vi "CheckAllPreferences.vi"() -> ()   [LabVIEW 2022 SP3]
uses:
  <vilib>/Utility/miscctls.llb/LVRangeTypeDef.ctl
  PreferencesControl.ctl
  Mic/Mic_Global.vi
panel:
  in  "Tab Control":enum32{"Files", "Globlals"}(tab)
  out "description":string
  out "Test Globals":T1
  out "Notes Out":string
  out "DataPath Out":path
  in  "Lists":u16(ring) items=["favorites", "117 vlns by B1 avg HV", "Admittance repeatability", "All 123 vlns group avg", "Internal mic 20920 ", "IVCI 18 all H adm rad", "ivci18 top 13 Adm H.AvR", "IVCI18 top 13 rad. H avg", "Mic distance B", "Mic distance test H12", "New York HV", "Paris 12 HV", "Rubio 6 spherical equatorial", "Some favorites 2018-2021", "String tension experiment", "Violas"]
  out "FRF settings":cluster{"XScale.Range":T2, "YScale.Range":T2}
  out "View":T3={"Alerts"=FALSE, "Log X Axis"=TRUE, "dB scale"=TRUE, "Averaging"=TRUE, "Fade"=0.8181818181818182, "Centroids?"=TRUE, "line thickness"=1}
  out "X Settings":cluster{"X_Low":dbl, "X_High":dbl}
  out "List contents":string
  in  "Templates":u16(ring) items=["", "accelerometer taptone Scratchpad", "Admittance H", "Admittance Scratchpad", "Current Settings", "Internal mic H", "JC Admit H laser", "JC Admit.HV laser", "JC H 12 radiation", "JC H 7 radiation", "JC HV 24 radiation", "Laser Admitance ScratchPad", "Radiation H 1", "Radiation ScratchPad", "ScratchPad", "Tap repeatabilty H20", "TapTones ScratchPad"]
  out "Settings out":T4={"Name of test"="", "Date"=timestamp(0 s since 1904-01-01), "Location"="", "Template"="", "Soundcard"="", "resolution"=32, "Sampling rate"=48000, "Ch1 Gain "=25.0, "Ch2 Gain"=10.0, "Sample time (s)"=0.3, "Pre-trigger (s)"=0.01, "Hammer Threshold"=10.0, "Positions"=12, "Taps/Position"=5, "Set Names"="", "Freq resolution"=10.0, "Hammer cutoff"=0.0, "Mic cutoff"=0.0, "Double bounce "=0.0, "Hammer Cal"=10.0, "dB Offset"=0.0, "Accel Cal"=10.0, "Vibrometer Cal"=0.0, "Mic Cal"=0.0, "Output"=2, "Voltage Cal"=1.0, "Vibrometer Port"="ASRL27::INSTR", "Range"=4, "High Pass"=2, "Bandwidth"=4, "X Range"=[], "Y Range"=[], "dB Spread"=0.0, "Trigger"=0, "Ch_1"=25, "Ch_2"=25, "flip?"=FALSE, "60Hz"=FALSE, "Time offset"=0.0, "Piezo Cal"=1.0, "Default Notes"=""} {"Ch_2" min=1 step=1; "Ch_1" min=1 max=100 step=1; "Trigger" items=["Hammer (force)", "Self-tap", "Spacebar"]; "Bandwidth" items=["1 kHz"=1, "5 kHz"=5, "10 kHz"=10, "25 kHz"=25, "50 kHz"=50, "100 kHz"=100]; "High Pass" items=["Off", "13 Hz", "104 Hz"]; "Range" items=["10 mm/s"=1, "20 mm/s"=2, "50 mm/s"=5, "100 mm/s"=10, "200 mm/s"=20, "500 mm/s"=50, "1 m/s"=100, "2 m/s"=200]; "Output" items=["Accelerometer", "Speed (from acceleration)", "Microphone", "Vibrometer", "Piezo"]; "Voltage Cal" format="%#_13g"; "Ch2 Gain" format="%#_13g"; "Ch1 Gain" format="%#_13g"; "Double bounce" min=0.0; "Mic cutoff" min=0.0 format="%#_4g"; "Hammer cutoff" min=0.0 format="%#_4g"; "Freq resolution" min=0.0; "Pre-trigger (s)" format="%#_13g"; "Date" format="%<%H:%M\n%d/%m/%y>T"; "resolution" items=["16 bit"=16, "24 bit"=24, "32 bit"=32]; "Sampling rate" items=["22050 samp/s"=22050, "44100 samp/s"=44100, "48000 samp/s"=48000]}
  out "comma?":bool
  in  "Cal File":path
  out "DAQ":string="DAQX"
  out "Scratch":string="ScratchPad"
  out "ID":i32[](array[numeric])
  out "View 2":T3={"Alerts"=FALSE, "Log X Axis"=TRUE, "dB scale"=TRUE, "Averaging"=TRUE, "Fade"=0.8181818181818182, "Centroids?"=TRUE, "line thickness"=1}
  out "Version":string="ObieApp 1.1b3"
  out "Settings":T4={"Name of test"="", "Date"=timestamp(3691169924 s since 1904-01-01), "Location"="", "Template"="", "Soundcard"="", "resolution"=32, "Sampling rate"=48000, "Ch1 Gain "=25.0, "Ch2 Gain"=10.0, "Sample time (s)"=0.3, "Pre-trigger (s)"=0.01, "Hammer Threshold"=0.1, "Positions"=12, "Taps/Position"=5, "Set Names"="", "Freq resolution"=1.0, "Hammer cutoff"=0.0, "Mic cutoff"=0.0, "Double bounce "=0.1, "Hammer Cal"=23.6, "dB Offset"=0.0, "Accel Cal"=1.014, "Vibrometer Cal"=1.0, "Mic Cal"=48.5, "Output"=2, "Voltage Cal"=3.8, "Vibrometer Port"="ASRL27::INSTR", "Range"=50, "High Pass"=2, "Bandwidth"=25, "X Range"=[], "Y Range"=[], "dB Spread"=40.0, "Trigger"=0, "Ch_1"=1, "Ch_2"=2, "flip?"=FALSE, "60Hz"=FALSE, "Time offset"=0.0, "Piezo Cal"=1.0, "Default Notes"=""} {"Ch_2" min=1 step=1; "Ch_1" min=1 max=100 step=1; "Trigger" items=["Hammer (force)", "Self-tap", "Spacebar"]; "Bandwidth" items=["1 kHz"=1, "5 kHz"=5, "10 kHz"=10, "25 kHz"=25, "50 kHz"=50, "100 kHz"=100]; "High Pass" items=["Off", "13 Hz", "104 Hz"]; "Range" items=["10 mm/s"=1, "20 mm/s"=2, "50 mm/s"=5, "100 mm/s"=10, "200 mm/s"=20, "500 mm/s"=50, "1 m/s"=100, "2 m/s"=200]; "Output" items=["Accelerometer", "Speed (from acceleration)", "Microphone", "Vibrometer", "Piezo"]; "Voltage Cal" format="%#_13g"; "Ch2 Gain" format="%#_13g"; "Ch1 Gain" format="%#_13g"; "Double bounce" min=0.0; "Mic cutoff" min=0.0 format="%#_4g"; "Hammer cutoff" min=0.0 format="%#_4g"; "Freq resolution" min=0.0; "Pre-trigger (s)" format="%#_13g"; "Date" format="%<%H:%M\n%d/%m/%y>T"; "resolution" items=["16 bit"=16, "24 bit"=24, "32 bit"=32]; "Sampling rate" items=["22050 samp/s"=22050, "44100 samp/s"=44100, "48000 samp/s"=48000]}
  out "Default Settings":T4={"Name of test"="ScratchPad", "Date"=timestamp(0 s since 1904-01-01), "Location"="Home", "Template"="ScratchPad", "Soundcard"="OCTA-CAPTURE", "resolution"=32, "Sampling rate"=48000, "Ch1 Gain "=20.0, "Ch2 Gain"=20.0, "Sample time (s)"=0.3, "Pre-trigger (s)"=0.001, "Hammer Threshold"=0.01, "Positions"=12, "Taps/Position"=5, "Set Names"="H,V", "Freq resolution"=1.0, "Hammer cutoff"=0.025, "Mic cutoff"=0.25, "Double bounce "=0.01, "Hammer Cal"=1.0, "dB Offset"=0.0, "Accel Cal"=1.0, "Vibrometer Cal"=1.0, "Mic Cal"=1.0, "Output"=2, "Voltage Cal"=1.0, "Vibrometer Port"="ASRL27::INSTR", "Range"=50, "High Pass"=2, "Bandwidth"=25, "X Range"=[{"Minimum"=200.0, "Maximum"=10000.0, "Increment"=2500.0, "Minor Increment"=500.0, "Start"=2500.0}, {"Minimum"=0.0, "Maximum"=0.05, "Increment"=0.025, "Minor Increment"=0.0025, "Start"=0.0}, {"Minimum"=0.0, "Maximum"=0.3, "Increment"=0.1, "Minor Increment"=0.01, "Start"=0.0}, {"Minimum"=200.0, "Maximum"=10000.0, "Increment"=10.0, "Minor Increment"=100.0, "Start"=1000.0}], "Y Range"=[{"Minimum"=-25.0, "Maximum"=0.0, "Increment"=5.0, "Minor Increment"=1.0, "Start"=-25.0}, {"Minimum"=-0.1, "Maximum"=1.0, "Increment"=0.25, "Minor Increment"=0.05, "Start"=0.0}, {"Minimum"=-1.0, "Maximum"=1.0, "Increment"=0.5, "Minor Increment"=0.1, "Start"=-1.0}, {"Minimum"=-10.0, "Maximum"=30.0, "Increment"=10.0, "Minor Increment"=0.5, "Start"=-10.0}], "dB Spread"=40.0, "Trigger"=0, "Ch_1"=1, "Ch_2"=2, "flip?"=FALSE, "60Hz"=FALSE, "Time offset"=0.0, "Piezo Cal"=1.0, "Default Notes"=""} {"Ch_2" min=1 step=1; "Ch_1" min=1 max=100 step=1; "Trigger" items=["Hammer (force)", "Self-tap", "Spacebar"]; "Bandwidth" items=["1 kHz"=1, "5 kHz"=5, "10 kHz"=10, "25 kHz"=25, "50 kHz"=50, "100 kHz"=100]; "High Pass" items=["Off", "13 Hz", "104 Hz"]; "Range" items=["10 mm/s"=1, "20 mm/s"=2, "50 mm/s"=5, "100 mm/s"=10, "200 mm/s"=20, "500 mm/s"=50, "1 m/s"=100, "2 m/s"=200]; "Output" items=["Accelerometer", "Speed (from acceleration)", "Microphone", "Vibrometer", "Piezo"]; "Voltage Cal" format="%#_13g"; "Ch2 Gain" format="%#_13g"; "Ch1 Gain" format="%#_13g"; "Double bounce" min=0.0; "Mic cutoff" min=0.0 format="%#_4g"; "Hammer cutoff" min=0.0 format="%#_4g"; "Freq resolution" min=0.0; "Pre-trigger (s)" format="%#_13g"; "Date" format="%<%H:%M\n%d/%m/%y>T"; "resolution" items=["16 bit"=16, "24 bit"=24, "32 bit"=32]; "Sampling rate" items=["22050 samp/s"=22050, "44100 samp/s"=44100, "48000 samp/s"=48000]}
  in  "Last":path
  out "devices":string[](array[string])=["Built-in Microph", "OCTA-CAPTURE"]
  in  "Task":T5(ring)=enum."One Shot - waiting"
  # "Hz"
  # "dB"
  # "dB"
  # "sec"
  # "sec"
  # "mV/Pa"
  # "mV/m/s2"
  # "mV/mm/s"
  # "V/N"
  # "sec"
  # "sec"
  # "mV/N"
  # "a.u."
  # "a.u."
  # "sec"
  # "Microphone"
  # "Labels"
  # "File Info"
  # "Hz"
  # "dB"
  # "dB"
  # "sec"
  # "sec"
  # "mV/Pa"
  # "mV/m/s2"
  # "mV/mm/s"
  # "V/N"
  # "sec"
  # "sec"
  # "mV/N"
  # "a.u."
  # "a.u."
  # "sec"
  # "Hz"
  # "dB"
  # "dB"
  # "sec"
  # "sec"
  # "mV/Pa"
  # "mV/m/s2"
  # "mV/mm/s"
  # "V/N"
  # "sec"
  # "sec"
  # "mV/N"
  # "a.u."
  # "a.u."
  # "sec"
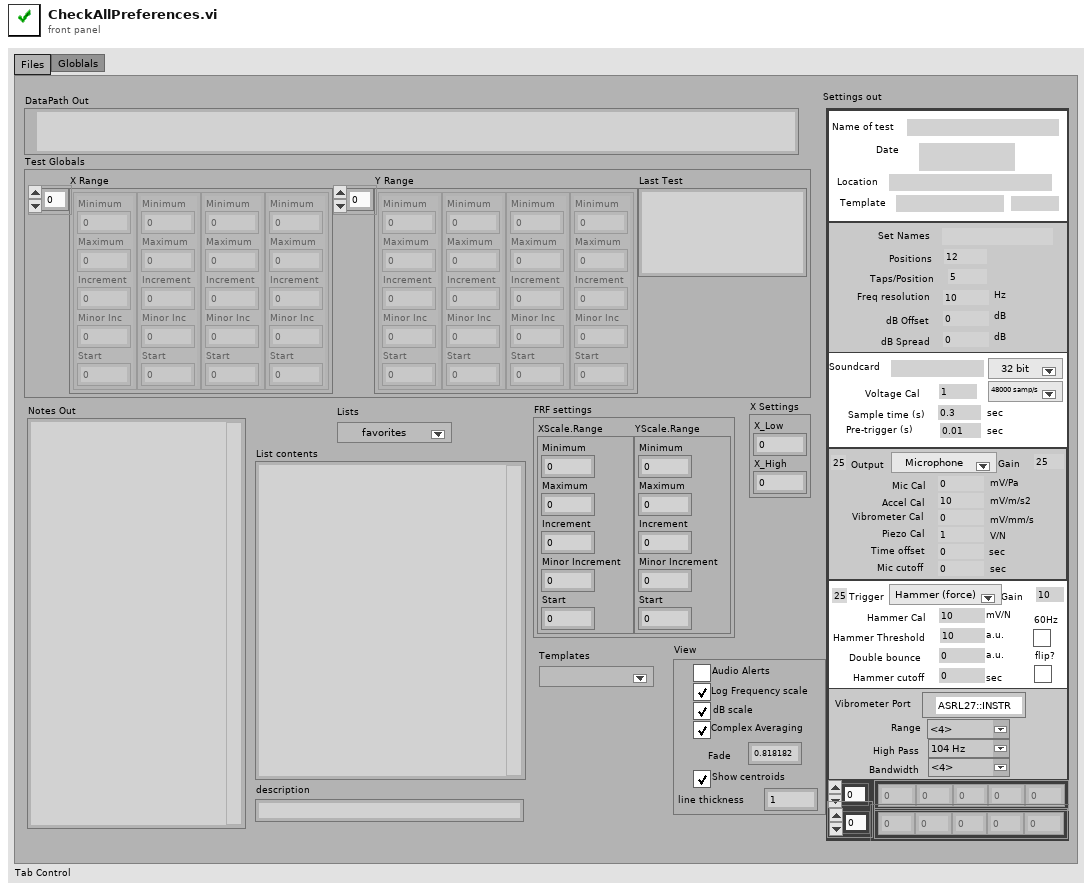
[diagram p1: front panel]
types:
  T1 = cluster{"X Range":cluster{"Minimum":dbl, "Maximum":dbl, "Increment":dbl, "Minor Inc":dbl, "Start":dbl}[], "Y Range":cluster{"Minimum":dbl, "Maximum":dbl, "Increment":dbl, "Minor Inc":dbl, "Start":dbl}[], "Last Test":string}
  T2 = typedef "LVRangeTypeDef.ctl" = cluster{"Minimum":dbl, "Maximum":dbl, "Increment":dbl, "Minor Increment":dbl, "Start":dbl}
  T3 = cluster{"Alerts":bool, "Log X Axis":bool, "dB scale":bool, "Averaging":bool, "Fade":dbl, "Centroids?":bool, "line thickness":u8}
  T4 = typedef "PreferencesControl.ctl" = cluster{"Name of test":string, "Date":timestamp, "Location":string, "Template":string, "Soundcard":string, "resolution":u16, "Sampling rate":u16, "Ch1 Gain ":dbl, "Ch2 Gain":dbl, "Sample time (s)":dbl, "Pre-trigger (s)":dbl, "Hammer Threshold":dbl, "Positions":i16, "Taps/Position":i16, "Set Names":string, "Freq resolution":dbl, "Hammer cutoff":dbl, "Mic cutoff":dbl, "Double bounce ":dbl, "Hammer Cal":dbl, "dB Offset":dbl, "Accel Cal":dbl, "Vibrometer Cal":dbl, "Mic Cal":dbl, "Output":u16, "Voltage Cal":dbl, "Vibrometer Port":refnum<visa-resource-name>, "Range":u16, "High Pass":u16, "Bandwidth":u16, "X Range":cluster{"Minimum":dbl, "Maximum":dbl, "Increment":dbl, "Minor Increment":dbl, "Start":dbl}[], "Y Range":cluster{"Minimum":dbl, "Maximum":dbl, "Increment":dbl, "Minor Increment":dbl, "Start":dbl}[], "dB Spread":dbl, "Trigger":u16, "Ch_1":u8, "Ch_2":u8, "flip?":bool, "60Hz":bool, "Time offset":dbl, "Piezo Cal":dbl, "Default Notes":string}
  T5 = enum16{"Initialize", "Free run", "One Shot - waiting", "One Shot - triggered", "Wait", "Close"}
  T6 = cluster{"X Range":T2[], "Y Range":T2[], "Last Test":string}
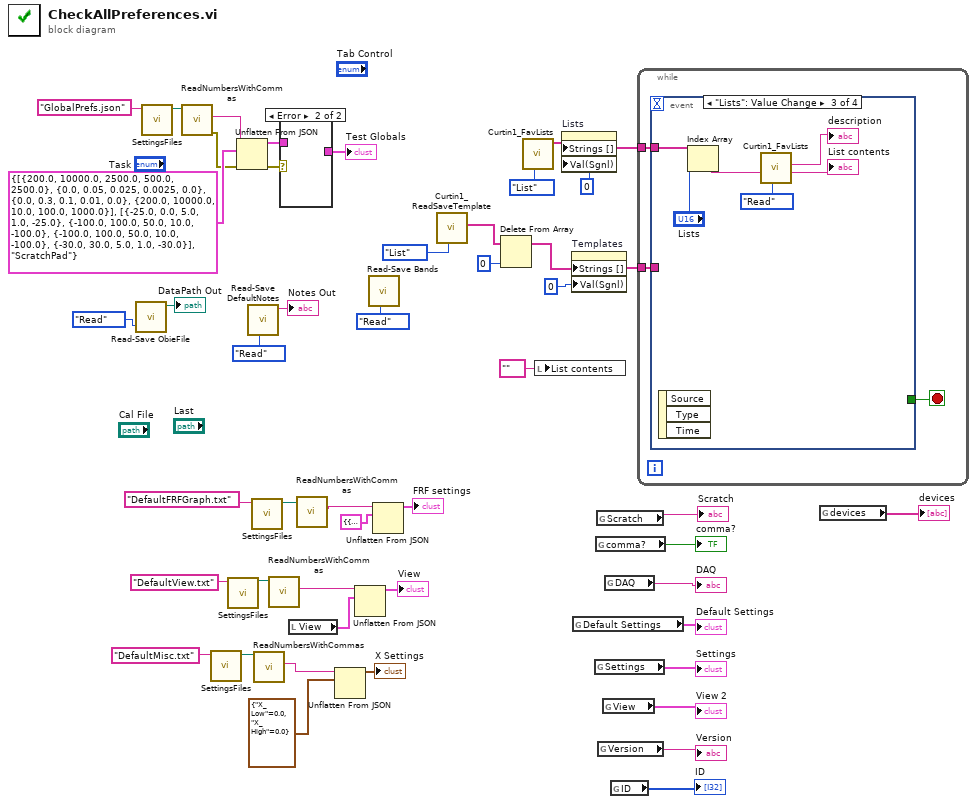
[diagram p0: block diagram]
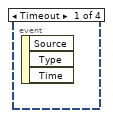
[diagram p2: hidden frame]
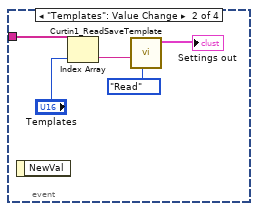
[diagram p3: hidden frame]
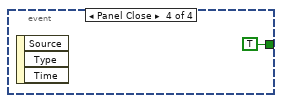
[diagram p4: hidden frame]
diagram:
  n1 = call "Read-Save ObieFile.vi"("Task"=enum16{"Save", "Read"}."Read") -> ("DataPath Out"=→"DataPath Out":path)  [unwired: 8 in, 2 out]
  n2 = call "SettingsFiles.vi"("settings file name"="GlobalPrefs.json" ("name or relative path")) -> ("file path"=w1:path)  [unwired: 9 in, 1 out]
  n3 = call "ReadNumbersWithCommas.vi"("file (use dialog)"=w1) -> ("error out"=w19:errorcluster, "text"=w18:string)  [unwired: 7 in, 2 out]
  n4 = call "SettingsFiles.vi"("settings file name"="DefaultMisc.txt" ("name or relative path")) -> ("file path"=w6:path)  [unwired: 9 in, 1 out]
  n5 = call "SettingsFiles.vi"("settings file name"="DefaultView.txt" ("name or relative path")) -> ("file path"=w3:path)  [unwired: 9 in, 1 out]
  n6 = Unflatten From JSON(JSON string=w18, type and defaults=T6 {"X Range"=[{"Minimum"=200.0, "Maximum"=10000.0, "Increment"=2500.0, "Minor Increment"=500.0, "Start"=2500.0}, {"Minimum"=0.0, "Maximum"=0.05, "Increment"=0.025, "Minor Increment"=0.0025, "Start"=0.0}, {"Minimum"=0.0, "Maximum"=0.3, "Increment"=0.1, "Minor Increment"=0.01, "Start"=0.0}, {"Minimum"=200.0, "Maximum"=10000.0, "Increment"=10.0, "Minor Increment"=100.0, "Start"=1000.0}], "Y Range"=[{"Minimum"=-25.0, "Maximum"=0.0, "Increment"=5.0, "Minor Increment"=1.0, "Start"=-25.0}, {"Minimum"=-100.0, "Maximum"=100.0, "Increment"=50.0, "Minor Increment"=10.0, "Start"=-100.0}, {"Minimum"=-100.0, "Maximum"=100.0, "Increment"=50.0, "Minor Increment"=10.0, "Start"=-100.0}, {"Minimum"=-30.0, "Maximum"=30.0, "Increment"=5.0, "Minor Increment"=1.0, "Start"=-30.0}], "Last Test"="ScratchPad"} ("Default"), error in (no error)=w19) -> (value=w45:T6, error out=w46:errorcluster)  [unwired: 4 in]
  n7 = call "Read-Save DefaultNotes.vi"("Task"=enum16{"Save", "Read"}."Read") -> ("Notes Out"=→"Notes Out":string)  [unwired: 9 in, 1 out]
  n8 = call "SettingsFiles.vi"("settings file name"="DefaultFRFGraph.txt" ("name or relative path")) -> ("file path"=w7:path)  [unwired: 9 in, 1 out]
  n9 = call "ReadNumbersWithCommas.vi"("file (use dialog)"=w6) -> ("text"=w22:string)  [unwired: 7 in, 3 out]
  n10 = call "ReadNumbersWithCommas.vi"("file (use dialog)"=w3) -> ("text"=w20:string)  [unwired: 7 in, 3 out]
  n11 = case shown="Error" w46 {
    tunnel: [w47 _] -> w43
    tunnel: w45 -> [w47 _]
    frame No Error {
    }
    frame Error {
    }
  }
  "Test Globals" <- w43
  n12 = local read "View"() -> (w32:T3)
  n13 = call "ReadNumbersWithCommas.vi"("file (use dialog)"=w7) -> ("text"=w21:string)  [unwired: 7 in, 3 out]
  n14 = Unflatten From JSON(JSON string=w22, type and defaults=cluster{"X_Low":dbl, "X_High":dbl} {"X_Low"=0.0, "X_High"=0.0} ("output cluster")) -> (value=→"X Settings":cluster{"X_Low":dbl, "X_High":dbl})  [unwired: 5 in, 1 out]
  n15 = Unflatten From JSON(JSON string=w20, type and defaults=w32) -> (value=→"View":T3)  [unwired: 5 in, 1 out]
  n16 = call "Read-Save Bands.vi"("Task"=enum16{"Save", "Read", "List"}."Read") -> ()  [unwired: 7 in, 4 out]
  n17 = Unflatten From JSON(JSON string=w21, type and defaults=cluster{"XScale.Range":T2, "YScale.Range":T2} {"XScale.Range"={"Minimum"=0.0, "Maximum"=0.0, "Increment"=0.0, "Minor Increment"=0.0, "Start"=0.0}, "YScale.Range"={"Minimum"=0.0, "Maximum"=0.0, "Increment"=0.0, "Minor Increment"=0.0, "Start"=0.0}} ("output cluster")) -> (value=→"FRF settings":cluster{"XScale.Range":T2, "YScale.Range":T2})  [unwired: 5 in, 1 out]
  n18 = call "Curtin1_ReadSaveTemplate.vi"("Task"=enum16{"Save", "Read", "List"}."List") -> ("List"=w24:string[])  [unwired: 7 in, 3 out]
  n19 = Delete From Array(array=w24, index=0) -> (array with subset deleted=w23:string[])  [unwired: 1 in, 1 out]
  n20 = call "Curtin1_FavLists.vi"("Task"=enum16{"Save", "Read", "List", "Delete"}."List") -> ("Lists"=w28:string[])  [unwired: 7 in, 3 out]
  n21 = local write "List contents"("" ("List contents")) -> ()
  n22 = property on="Lists" class="Ring (strict)"("Strings []"=w28, "Val(Sgnl)"=0) -> ()  [unwired: 2 in, 2 out]
  n23 = property on="Templates" class="Ring (strict)"("Strings []"=w23, "Val(Sgnl)"=0) -> ()  [unwired: 2 in, 2 out]
  n24 = global read "Mic_Global.vi" "Default Settings"() -> (→"Default Settings":T4)
  n25 = global read "Mic_Global.vi" "Settings"() -> (→"Settings":T4)
  n26 = global read "Mic_Global.vi" "comma?"() -> (→"comma?":bool)
  n27 = global read "Mic_Global.vi" "Scratch"() -> (→"Scratch":string)
  n28 = global read "Mic_Global.vi" "Version"() -> (→"Version":string)
  n29 = global read "Mic_Global.vi" "View"() -> (→"View 2":T3)
  n30 = global read "Mic_Global.vi" "DAQ"() -> (→"DAQ":string)
  n31 = global read "Mic_Global.vi" "ID"() -> (→"ID":i32[])
  n32 = while {
    tunnel: w23 -> [w50]
    tunnel: w28 -> [w49]
    stop <- w48 stop-if-true
    n33 = event shown="[2] \"Lists\": Value Change" {
      selector: _ -> [_ _ _ _]
      dyn-events: _ -> [_ _ _ _]
      timeout: _ -> [_ _ _ _]
      tunnel: w50 -> [_ w55 _ _]
      tunnel: w49 -> [_ _ w61 _]
      tunnel: [_ _ _ TRUE] -> w48
      event Timeout {
        n34 = event-data() -> ()  [unwired: 1 in, 3 out]
      }
      event "Templates": Value Change {
        n35 = event-data() -> ()  [unwired: 1 in, 1 out]
        n36 = Index Array(array=w55, index="Templates") -> (element=w53:string)
        n37 = call "Curtin1_ReadSaveTemplate.vi"("Task"=enum16{"Save", "Read", "List"}."Read", "Template"=w53) -> ("Settings out"=→"Settings out":T4)  [unwired: 6 in, 3 out]
      }
      event "Lists": Value Change {
        n38 = event-data() -> ()  [unwired: 1 in, 3 out]
        n39 = Index Array(array=w61, index="Lists") -> (element=w59:string)
        n40 = call "Curtin1_FavLists.vi"("Task"=enum16{"Save", "Read", "List", "Delete"}."Read", "List Name"=w59) -> ("String"=→"List contents":string, "description out"=→"description":string)  [unwired: 6 in, 2 out]
      }
      event Panel Close {
        n41 = event-data() -> ()  [unwired: 1 in, 3 out]
      }
    }
  }
  n42 = global read "Mic_Global.vi" "devices"() -> (→"devices":string[])
